vi "Set_Close_Method_Info.vi"(8 "expId":string) -> (3 "String":string)   [LabVIEW 2013]
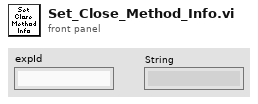
[diagram p1: front panel]
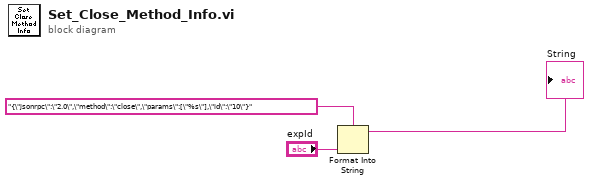
[diagram p0: block diagram]
diagram:
  n1 = Format Into String(format string="{\"jsonrpc\":\"2.0\",\"method\":\"close\",\"params\":[\"%s\"],\"id\":\"10\"}" ("input string"), "expId") -> (resulting string=→"String":string)  [unwired: 2 in, 1 out]
